vi "sts_calc_subvi.vi"(10 "Array 2":dbl[](array[numeric]), 11 "Array":dbl[](array[numeric])) -> (3 "STS":dbl)   [LabVIEW 2011]
uses:
  <vilib>/Analysis/NI_AALPro.lvlib
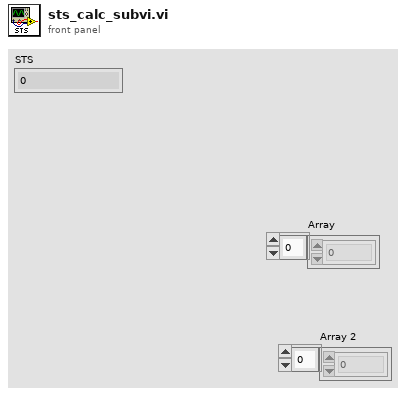
[diagram p1: front panel]
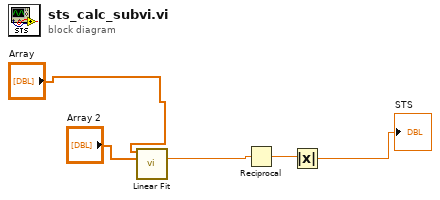
[diagram p0: block diagram]
diagram:
  n1 = call <vilib>:"Linear Fit.vi"("Y"="Array", "X"="Array 2") -> ("slope"=w4:dbl)  [unwired: 9 in, 4 out]
  n2 = Reciprocal(x=w4) -> (1/x=w2:dbl)
  n3 = Absolute Value(x=w2) -> (abs(x)=→"STS":dbl)
